vi "ToDatagram.vi"(8 "error in (no error)":errorcluster, 10 "messageID":u16, 11 "PublishAckMqttMsg in":refnum<class "PublishAckMqttMsg.lvclass">) -> (0 "error out":errorcluster, 2 "Datagram":u8[](array[numeric]), 3 "PublishAckMqttMsg out":refnum<class "PublishAckMqttMsg.lvclass">)   [LabVIEW 2020, in "PublishAckMqttMsg.lvclass"]
uses:
  PublishAckMqttMsg.lvclass
  mqttTypedef/mqttMessageType.ctl
  mqttTypedef/mqttQOSlevel.ctl
  PublishAckMqttMsg.lvclass/PublishAckMqttMsg.ctl
  BaseMqttMsg.lvclass
  MQTT Client.lvclass
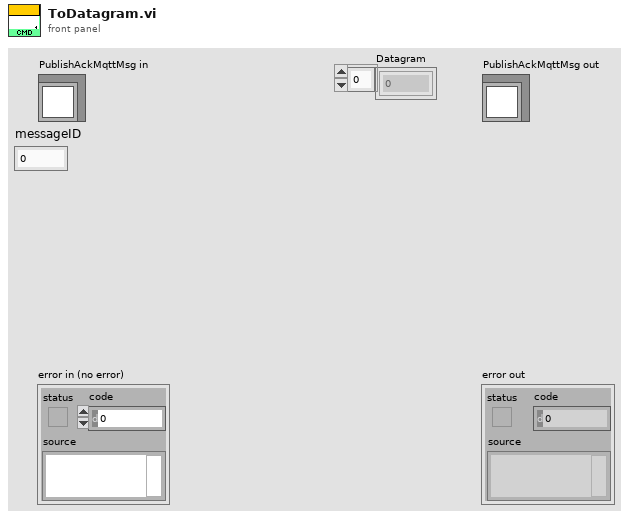
[diagram p1: front panel]
types:
  T1 = typedef "MQTT Client.lvclass/mqttQOSlevel.ctl" = enum8{"At most once", "At least once", "Exactly once", "Reserved"}
  T2 = typedef "MQTT Client.lvclass/mqttMessageType.ctl" = enum32{"Reserved", "CONNECT", "CONNACK", "PUBLISH", "PUBACK", "PUBREC", "PUBREL", "PUBCOMP", "SUBSCRIBE", "SUBACK", "UNSUBSCRIBE", "UNSUBACK", "PINGREQ", "PINGRESP", "DISCONNECT", "Reserved2"}
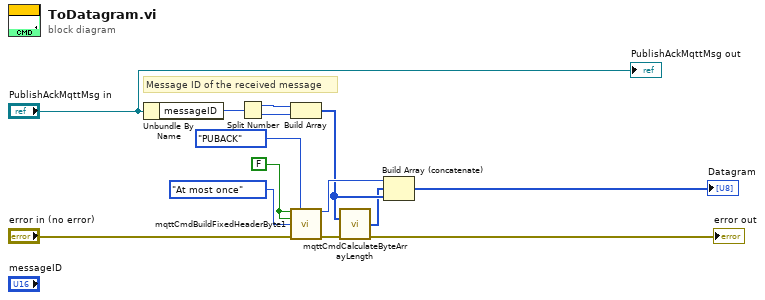
[diagram p0: block diagram]
diagram:
  w6 = FALSE ("retain(F)")
  # "Message ID of the received message"
  n1 = Unbundle By Name("PublishAckMqttMsg in") -> ("messageID"=w4:u16)
  n2 = Split Number(x=w4) -> (hi(x)=w10:u8, lo(x)=w11:u8)
  n3 = Build Array(w10, w11) -> (w9:u8[])
  n4 = call "mqttCmdBuildFixedHeaderByte1.vi"("retain(F)"=w6, "MessageType"=mqttMessageType."PUBACK", "duplicate(F)"=w6, "QoS (At most once)"=mqttQOSlevel."At most once", "error in (no error)"="error in (no error)") -> ("byte1"=w12:u8, "error out"=w8:errorcluster)  [unwired: 9 in]
  n5 = call "mqttCmdCalculateByteArrayLength.vi"("byteArry in"=w9, "error in (no error)"=w8) -> ("length out"=w7:u8[], "error out"=→"error out":errorcluster)  [unwired: 12 in]
  n6 = Build Array (concatenate)(w12, w7, w9) -> (→"Datagram":u8[])
  "PublishAckMqttMsg out" <- "PublishAckMqttMsg in"
